vi "tb_simio_host.vi"() -> ()   [LabVIEW 2010]
uses:
  <vilib>/Analysis/NI_AALBase.lvlib
panel:
  out "timed out?":bool
  in  "stop":bool
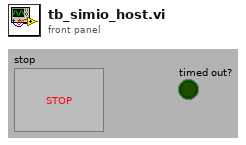
[diagram p1: front panel]
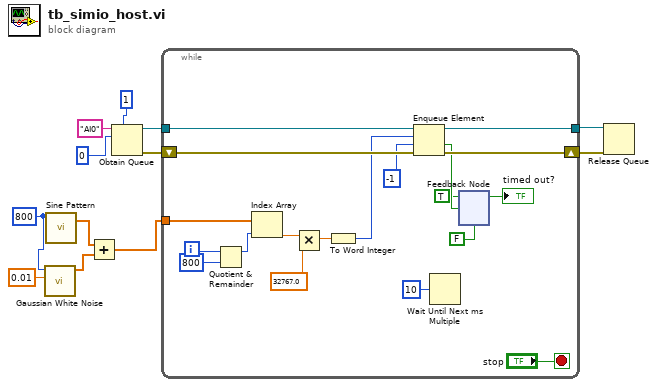
[diagram p0: block diagram]
diagram:
  w5 = 800 ("samples")
  n1 = call <vilib>:"Gaussian White Noise.vi"("standard deviation"=0.01, "samples"=w5) -> ("Gaussian noise pattern"=w3:dbl[])  [unwired: 8 in, 1 out]
  n2 = call <vilib>:"Sine Pattern.vi"("samples"=w5) -> ("Sinusoidal Pattern"=w4:dbl[])  [unwired: 3 in, 1 out]
  n3 = Add(x=w4, y=w3) -> (x+y=w2:dbl[])
  n4 = Obtain Queue(max queue size (-1, unlimited)=1, name (unnamed)="AI0", element data type=i16 0) -> (queue out=w10:refnum<queue>, error out=w8:errorcluster)  [unwired: 2 in, 1 out]
  n5 = while {
    tunnel: w10 -> [w31]
    shift-right: [w20] -> w6
    shift-left: w8 -> [w30]
    tunnel: w2 -> [w29]
    tunnel: [w21] -> w7
    i -> [w28]
    stop <- "stop" stop-if-true
    n6 = Quotient & Remainder(x=w28, y=800) -> (x-y*floor(x/y)=w26:i32)  [unwired: 1 out]
    n7 = Index Array(array=w29, index=w26) -> (element=w25:dbl)
    n8 = Multiply(x=w25, y=32767.0) -> (x*y=w23:dbl)
    n9 = To Word Integer(number=w23) -> (16bit integer=w22:i16)
    n10 = Enqueue Element(queue=w31, element=w22, timeout in ms (-1)=-1, error in (no error)=w30) -> (queue out=w21:refnum<queue>, timed out?=w16:bool, error out=w20:errorcluster)
    n11 = Wait Until Next ms Multiple(millisecond multiple=u32 10) -> ()  [unwired: 1 out]
    n12 = feedback-in #1(TRUE, w16) -> ()
    n13 = feedback #1(FALSE) -> (→"timed out?":bool)
  }
  n14 = Release Queue(queue=w7, error in (no error)=w6) -> ()  [unwired: 1 in, 3 out]
